vi "Save Picture to File.vi"(4 "Background Color":u32(colorbox)=16777215, 6 "depth":i32=24, 7 "Image Format":enum16{"JPEG", "PNG", "BMP"}(ring), 8 "error in (no error)":errorcluster, 9 "rect":T1, 10 "Image (Empty Picture)":picture, 11 "path (empty prompts)":path) -> (0 "error out":errorcluster, 3 "path out":path)   [LabVIEW 2011]
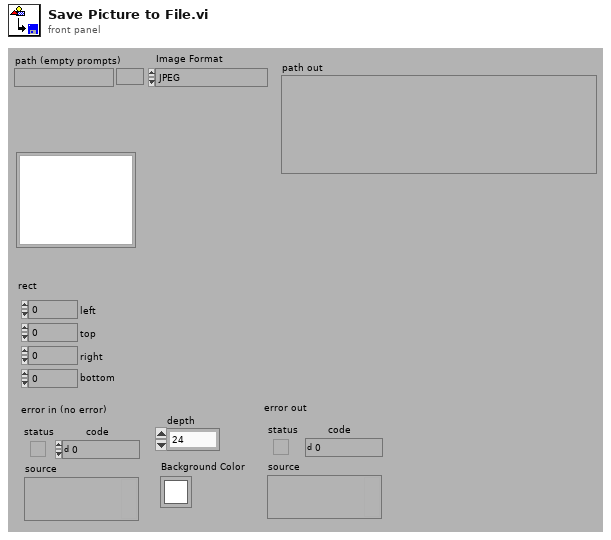
[diagram p1: front panel]
types:
  T1 = cluster{"left":i16, "top":i16, "right":i16, "bottom":i16}
  T2 = typedef "imagedata.ctl" = cluster{"image type":i32, "image depth":i32, "image":u8[], "mask":u8[], "colors":u32[], "Rectangle":cluster{"left":i16, "top":i16, "right":i16, "bottom":i16}}
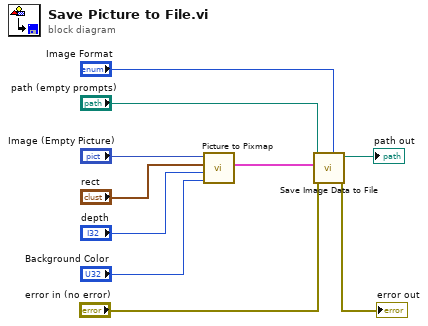
[diagram p0: block diagram]
diagram:
  n1 = call <vilib>:"Picture to Pixmap.vi"("Background Color"="Background Color", "depth"="depth", "rect"="rect", "picture"="Image (Empty Picture)") -> ("image data"=w4:T2)  [unwired: 7 out]
  n2 = call "Save Image Data to File.vi"("Image Format"="Image Format", "error in (no error)"="error in (no error)", "image data"=w4, "Path"="path (empty prompts)") -> ("error out"=→"error out":errorcluster, "Path Out"=→"path out":path)  [unwired: 1 in, 5 out]
